vi "Write VIA.vi"(8 "error in (no error)":errorcluster, 10 "VIA":string, 11 "Resource In":refnum<class "Resource.lvclass">) -> (0 "error out":errorcluster, 3 "Resource":refnum<class "Resource.lvclass">)   [LabVIEW 2020, in "RP2040.lvlib" / "RP2040Platform.lvclass"]
uses:
  RP2040Platform.lvclass
  Builds/picoG/ppl/PicoG-Core.lvlibp/PicoG-Processor/PicoG-Core/Resource/Resource.lvclass
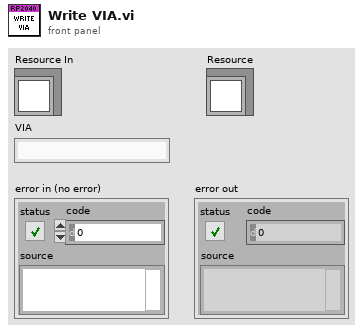
[diagram p1: front panel]
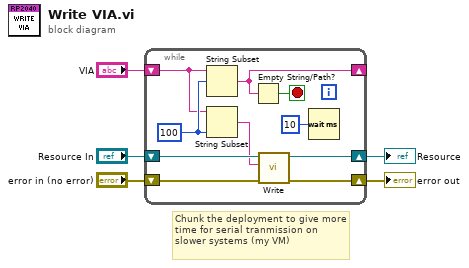
[diagram p0: block diagram]
diagram:
  # "Chunk the deployment to give more time for serial tranmission on slower systems (my VM)"
  n1 = while {
    shift-right: [w15] -> w5
    shift-left: "error in (no error)" -> [w14]
    shift-right: [w12] -> w2
    shift-left: "Resource In" -> [w13]
    shift-right: [w7] -> _
    shift-left: "VIA" -> [w9]
    stop <- w6 stop-if-true
    w10 = 100 ("length (rest)")
    n2 = String Subset(string=w9, offset (0)=w10) -> (substring=w7:string)  [unwired: 1 in]
    n3 = String Subset(string=w9, length (rest)=w10) -> (substring=w8:string)  [unwired: 1 in]
    n4 = Empty String/Path?(string/path=w7) -> (empty?=w6:bool)
    n5 = call "Write.vi"("error in (no error)"=w14, "Data"=w8, "DeployResource in"=w13) -> ("error out"=w15:errorcluster, "DeployResource out"=w12:refnum<class "Resource.lvclass">)  [unwired: 6 in, 1 out]
    n6 = Wait (ms)(milliseconds to wait=u32 10) -> ()  [unwired: 1 out]
  }
  "Resource" <- w2
  "error out" <- w5
